vi "Length Hex.vi"(0 "Bytes in":u8[](array[numeric]), 7 "Length":i32, 11 "Start Index(0)":i32) -> (4 "Remaining Bytes out":u8[](array[numeric]), 6 "Hex Bytes":u8[](array[numeric]), 8 "Hex string":string, 10 "Hex number":u64, 15 "End Index":i32)   [LabVIEW 2014, in "hse-db.lvlib" / "MySQL (TCP).lvlib"]
uses:
  MySQL (TCP).lvlib
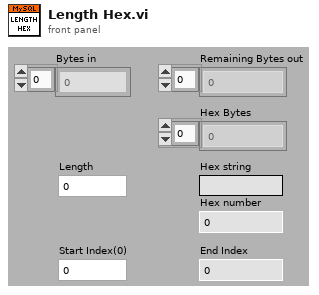
[diagram p1: front panel]
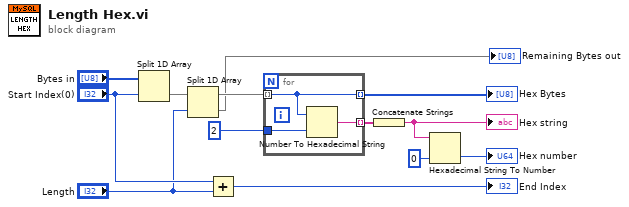
[diagram p0: block diagram]
diagram:
  n1 = Split 1D Array(array="Bytes in", index="Start Index(0)") -> (second subarray=w5:u8[])  [unwired: 1 out]
  n2 = Split 1D Array(array=w5, index="Length") -> (first subarray=w3:u8[], second subarray=→"Remaining Bytes out":u8[])
  n3 = Add(x="Start Index(0)", y="Length") -> (x+y=→"End Index":i32)
  n4 = for {
    tunnel: [w16] -> w13 mode=indexing
    tunnel: i16 2 ("width (-)") -> [w15]
    tunnel: w3 -> [w14] mode=indexing
    tunnel: [w14] -> w1 mode=indexing
    n5 = Number To Hexadecimal String(1:w15, 2:w14) -> (0:w16:string)
  }
  "Hex Bytes" <- w1
  n6 = Concatenate Strings(w13) -> (w11:string)
  "Hex string" <- w11
  n7 = Hexadecimal String To Number(string=w11, default (0uL)=u64 0 ("default (0 U32)")) -> (number=→"Hex number":u64)  [unwired: 1 in, 1 out]
